vi "analyse_range.vi"(0 "X search min (/cm)":sgl, 1 "X search max (/cm)":sgl, 4 "X min":sgl, 5 "X max":sgl, 7 "full range":bool, 9 "length":u32) -> (14 "index start":u32, 15 "index stop":u32)   [LabVIEW 2010, in "OSA.lvclass"]
uses:
  OSA.lvclass
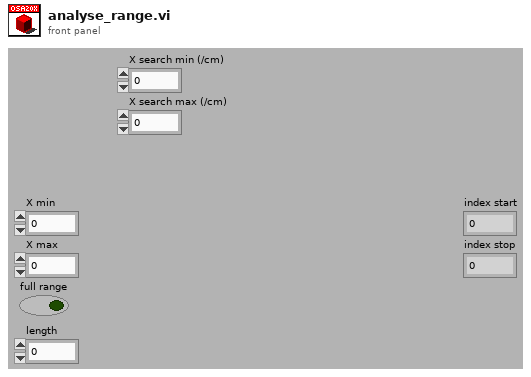
[diagram p1: front panel]
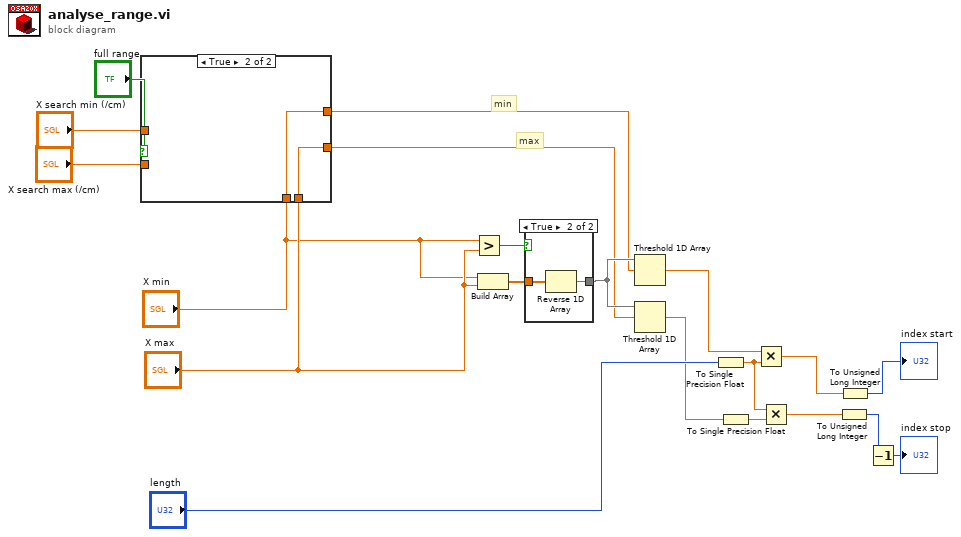
[diagram p0: block diagram]
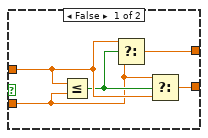
[diagram p3: hidden frame]
diagram:
  # "max"
  # "min"
  n1 = case shown="True" "full range" {
    tunnel: [w25 w27] -> w9
    tunnel: "X search min (/cm)" -> [w24 _]
    tunnel: "X search max (/cm)" -> [w22 _]
    tunnel: [w21 w26] -> w8
    tunnel: "X min" -> [_ w27]
    tunnel: "X max" -> [_ w26]
    frame False {
      n2 = Less Or Equal?(x=w24, y=w22) -> (x <= y?=w23:bool)
      n3 = Select(t=w24, s=w23, f=w22) -> (s? t:f=w25:sgl)
      n4 = Select(t=w22, s=w23, f=w24) -> (s? t:f=w21:sgl)
    }
    frame True {
    }
  }
  n5 = Greater?(x="X min", y="X max") -> (0:w14:bool)
  n6 = Build Array("X min", "X max") -> (w15:sgl[])
  n7 = case shown="True" w14 {
    tunnel: w15 -> [w28 w30]
    tunnel: [w28 w29] -> w13
    frame False {
    }
    frame True {
      n8 = Reverse 1D Array(array=w30) -> (reversed array=w29:sgl[])
    }
  }
  n9 = Threshold 1D Array(2:w9, 3:w13) -> (0:w12:sgl)  [unwired: 1 in]
  n10 = Threshold 1D Array(2:w8, 3:w13) -> (0:w6:sgl)  [unwired: 1 in]
  n11 = To Single Precision Float(number="length") -> (single precision float=w2:sgl)
  n12 = To Single Precision Float(number=w6) -> (single precision float=w20:sgl)
  n13 = Multiply(x=w12, y=w2) -> (x*y=w5:sgl)
  n14 = Multiply(x=w2, y=w20) -> (x*y=w19:sgl)
  n15 = To Unsigned Long Integer(number=w19) -> (unsigned 32bit integer=w3:u32)
  n16 = To Unsigned Long Integer(number=w5) -> (unsigned 32bit integer=→"index start":u32)
  n17 = Decrement(x=w3) -> (x-1=→"index stop":u32)
